vi "Get Name.vi"(11 "Thread in":refnum<class "Thread.lvclass">) -> (2 "name":string, 3 "Thread out":refnum<class "Thread.lvclass">)   [LabVIEW 2019, in "DSF Core.lvlib" / "Thread.lvclass"]
uses:
  Thread.lvclass
  Thread.lvclass/Thread.ctl
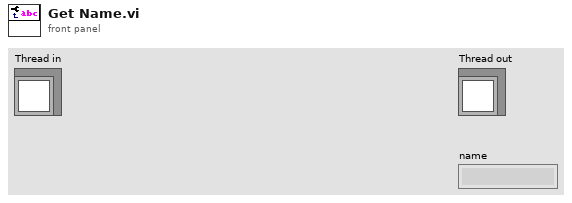
[diagram p1: front panel]
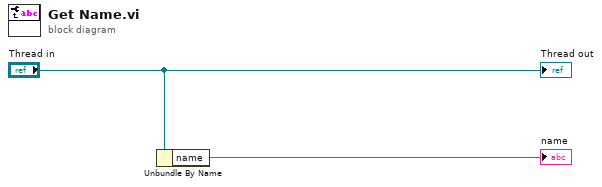
[diagram p0: block diagram]
diagram:
  n1 = Unbundle By Name("Thread in") -> ("name"=→"name":string)
  "Thread out" <- "Thread in"
